vi "Get Palette Names.vi"(7 "Run Mode?":bool, 8 "error in (no error)":errorcluster, 9 "Visibility":T1, 10 "3D Plot.lvclass in":refnum<class "3D Plot.lvclass">, 11 "MenuRef":refnum<k9>) -> (0 "error out":errorcluster, 2 "3D Plot.lvclass out":refnum<class "3D Plot.lvclass">, 3 "Dup MenuRef":refnum<k9>)   [LabVIEW 2017, in "3D Plot.lvclass"]
uses:
  <vilib>/Math Plots/3D Math Plots/3D Plot/3D Plot/3D Plot.lvclass
  <vilib>/Math Plots/3D Math Plots/3D Plot/3D Plot/Typedef/Item Visibility.ctl
panel:
  in  "Visibility Item Names":string[](array[string])=["", "Projection Palette", "Color Ramp"]
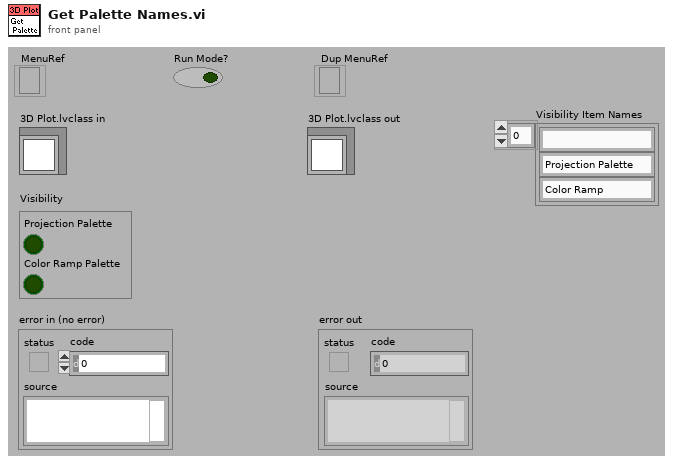
[diagram p1: front panel]
types:
  T1 = typedef "3D Plot.lvclass/Item Visibility.ctl" = cluster{"Projection Palette":bool, "Color Ramp Palette":bool}
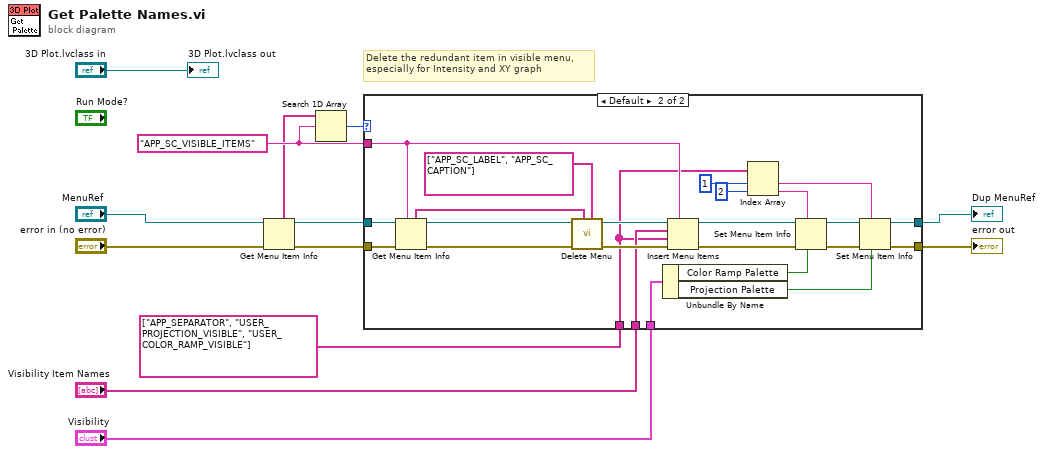
[diagram p0: block diagram]
diagram:
  w13 = "APP_SC_VISIBLE_ITEMS"
  # "Delete the redundant item in visible menu, \nespecially for Intensity and XY graph"
  n1 = Get Menu Item Info(8:"error in (no error)", 11:"MenuRef") -> (0:w7:errorcluster, 3:w9:refnum<k9>, 5:w8:string[])  [unwired: 5 out]
  n2 = Search 1D Array(1D array=w8, element=w13) -> (index of element=w12:i32)  [unwired: 1 out]
  n3 = case shown="Default" w12 {
    tunnel: w9 -> [w15 w39]
    tunnel: [w15 w19] -> w11
    tunnel: w7 -> [w14 w38]
    tunnel: [w14 w16] -> w1
    tunnel: w13 -> [_ w34]
    tunnel: "Visibility" -> [_ w36]
    tunnel: "Visibility Item Names" -> [_ w18]
    tunnel: string[] ["APP_SEPARATOR", "USER_PROJECTION_VISIBLE", "USER_COLOR_RAMP_VISIBLE"] ("item names") -> [_ w17]
    frame -1 {
    }
    frame Default {
      n4 = Get Menu Item Info(7:w34, 8:w38, 11:w39) -> (0:w24:errorcluster, 3:w25:refnum<k9>, 5:w21:string[])  [unwired: 4 out]
      n5 = call <vilib>:"Delete Menu.vi"("Submenu Tags Validated"=string[] ["APP_SC_LABEL", "APP_SC_CAPTION"], "Submenu Tags to Check"=w21, "error in (no error)"=w24, "MenuRef"=w25) -> ("error out"=w22:errorcluster, "Dup MenuRef"=w23:refnum<k9>)  [unwired: 6 in]
      n6 = Unbundle By Name(w36) -> ("Color Ramp Palette"=w27:bool, "Projection Palette"=w26:bool)
      n7 = Insert Menu Items(5:w34, 6:w22, 7:w17, 8:w18, 9:w23) -> (0:w37:errorcluster, 3:w35:refnum<k9>)  [unwired: 2 out]
      n8 = Index Array(array=w17, index #1=1 ("index"), index #2=2 ("index")) -> (element #1=w31:string, element #2=w30:string)
      n9 = Set Menu Item Info(6:w27, 7:w30, 8:w37, 11:w35) -> (0:w33:errorcluster, 3:w32:refnum<k9>)  [unwired: 3 out]
      n10 = Set Menu Item Info(6:w26, 7:w31, 8:w33, 11:w32) -> (0:w16:errorcluster, 3:w19:refnum<k9>)  [unwired: 3 out]
    }
  }
  "Dup MenuRef" <- w11
  "error out" <- w1
  "3D Plot.lvclass out" <- "3D Plot.lvclass in"
